vi "Account FGV Unit Testing.vi"() -> ()   [LabVIEW 2012]
uses:
  Account FGV/Account Methods.ctl
panel:
  out "账户余额":dbl
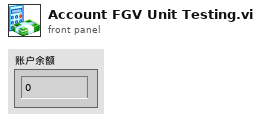
[diagram p1: front panel]
types:
  T1 = typedef "Account Methods.ctl" = enum16{"存款", "取款", "查询余额", "结清余额"}
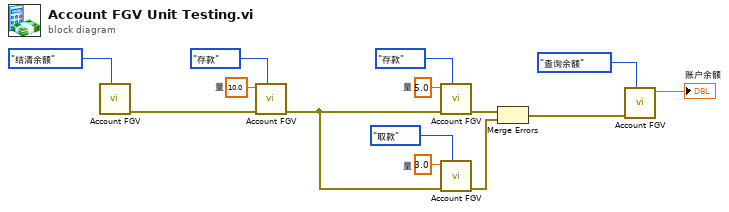
[diagram p0: block diagram]
diagram:
  w7 = 3.0  # 量
  w10 = 5.0  # 量
  w11 = 10.0  # 量
  n1 = call "Account FGV.vi"("账户方法"=Account_Methods."结清余额" ("银行命令")) -> ("错误输出"=w12:cluster{"状态":bool, "代码":i32, "源":string})  [unwired: 2 in, 8 out]
  n2 = call "Account FGV.vi"("账户方法"=Account_Methods."存款" ("银行命令"), "错误输入"=w12, "量"=w11) -> ("错误输出"=w4:cluster{"状态":bool, "代码":i32, "源":string})  [unwired: 8 out]
  n3 = call "Account FGV.vi"("账户方法"=Account_Methods."存款" ("银行命令"), "错误输入"=w4, "量"=w10) -> ("错误输出"=w3:cluster{"状态":bool, "代码":i32, "源":string})  [unwired: 8 out]
  n4 = call "Account FGV.vi"("账户方法"=Account_Methods."取款" ("银行命令"), "错误输入"=w4, "量"=w7) -> ("错误输出"=w2:cluster{"状态":bool, "代码":i32, "源":string})  [unwired: 8 out]
  n5 = Merge Errors ("合并错误")(w3, w2) -> (w1:errorcluster)
  n6 = call "Account FGV.vi"("账户方法"=Account_Methods."查询余额" ("银行命令"), "错误输入"=w1) -> ("账户余额"=→"账户余额":dbl)  [unwired: 1 in, 8 out]
